vi "3.90.2-Borrow FPGA Ref.vi"(4 "error in (no error)":errorcluster) -> (0 "error out":errorcluster, 1 "Failed to Obtain Ref":bool, 2 "element":T1, 3 "FPGA Ref":refnum<queue>)   [LabVIEW 2010]
doc: "Grabs a reference to the FPGA if it is not already in use. This reference is on a STRICT dequeue -lossy enqueue schedule because otherwise we might either duplicate or lose THE ONLY FPGA reference, which would be TRAGIC. Run the 3.90.3-Return FPGA Ref VI to cover your ass. DO NOT FORGET TO RUN THE 3.90.3 VI!"
uses:
  2-Low Neurons/2-FPGA VI Typedef.ctl
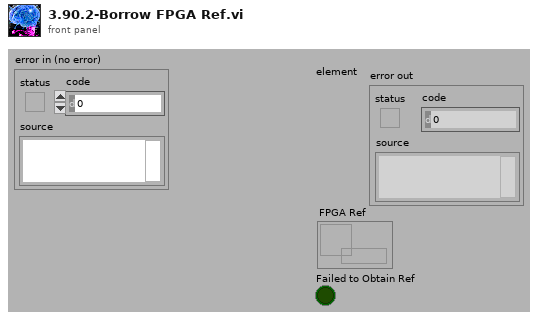
[diagram p1: front panel]
types:
  T1 = typedef "2-FPGA VI Typedef.ctl" = refnum<k20>
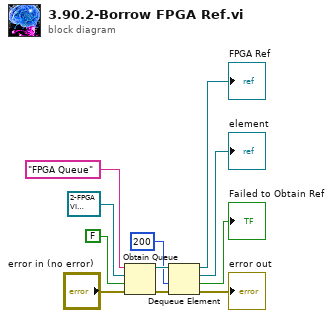
[diagram p0: block diagram]
diagram:
  n1 = Obtain Queue(name (unnamed)="FPGA Queue", element data type=T1 refnum ("FPGA VI Reference Out 2"), create if not found? (T)=FALSE, error in (no error)="error in (no error)") -> (queue out=w7:refnum<queue>, error out=w6:errorcluster)  [unwired: 1 in, 1 out]
  n2 = Dequeue Element(queue=w7, timeout in ms (-1)=200, error in (no error)=w6) -> (queue out=→"FPGA Ref":refnum<queue>, element=→"element":T1, timed out?=→"Failed to Obtain Ref":bool, error out=→"error out":errorcluster)
